vi "In Place_Unwired Terminals.vi"(8 "error in":errorcluster, 11 "In Place Node":refnum<vi>) -> (0 "error out":errorcluster, 1 "Unwired Indices For Removal":u32[](array[numeric]), 2 "Unwired Indices":u32[](array[numeric]), 3 "Output Terminals[]":refnum<vi>[](array[refnum]), 4 "Unwired?":bool[](array[boolean]))   [LabVIEW 2023]
doc: "Returns list of unwired terminals, and a separate list of those the can be removed. The latter will be different if all terminals are unwired, because you cannot remove *all* unwired terminals from the node.\n\nThe Unwired boolean array has one element per input/ouput terminal in inplace node."
panel:
  # "one element per terminal in node"
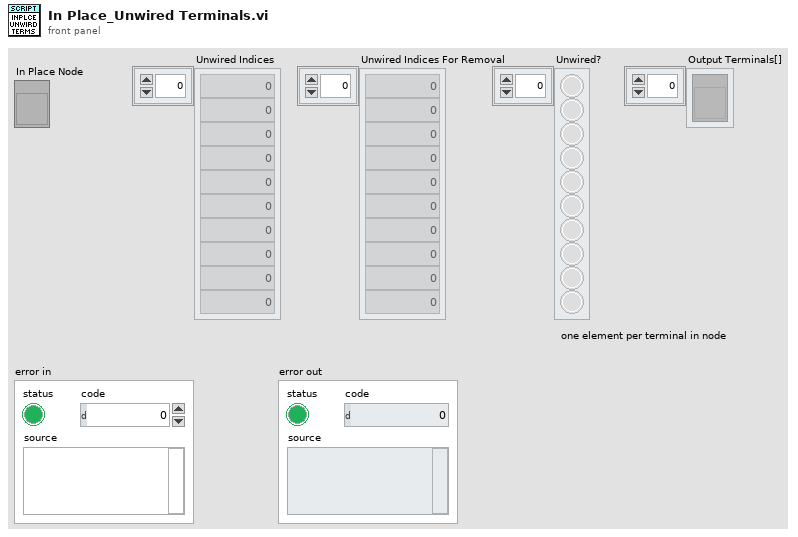
[diagram p1: front panel]
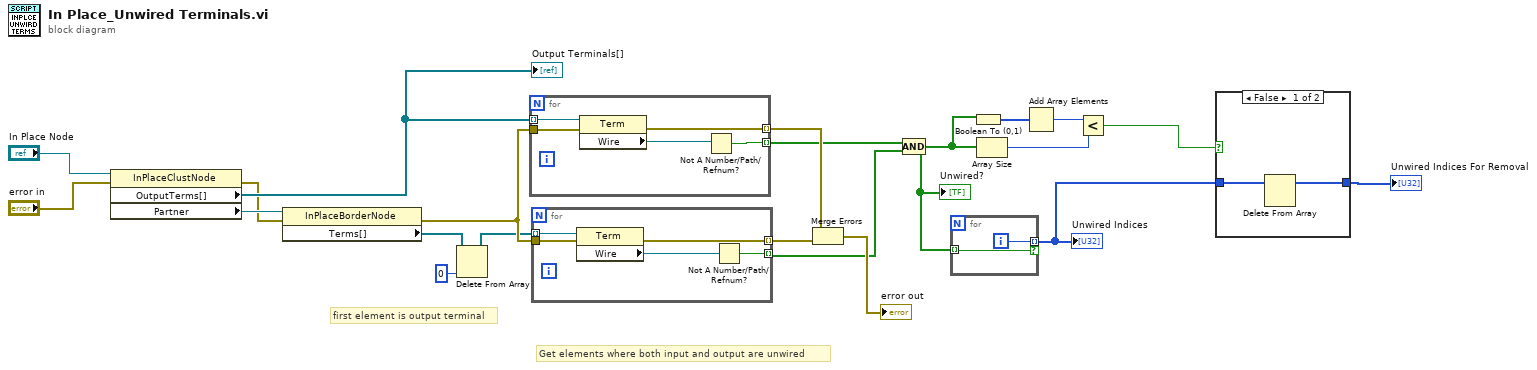
[diagram p0: block diagram]
diagram:
  # "first element is output terminal"
  # "Get elements where both input and output are unwired"
  n1 = property class="InPlaceClustNode"(reference="In Place Node", error in="error in") -> (error out=w15:errorcluster, "OutputTerms[]"=w19:refnum<vi>[], "Partner"=w21:refnum<vi>)  [unwired: 1 out]
  "Output Terminals[]" <- w19
  n2 = property class="InPlaceBorderNode"(reference=w21, error in=w15) -> (error out=w14:errorcluster, "Terms[]"=w5:refnum<vi>[])  [unwired: 1 out]
  n3 = Delete From Array(array=w5, index=0) -> (array with subset deleted=w4:refnum<vi>[])  [unwired: 1 in, 1 out]
  n4 = for {
    tunnel: [w22] -> w8 mode=indexing
    tunnel: w19 -> [w26] mode=indexing
    tunnel: w14 -> [w25]
    tunnel: [w24] -> w12 mode=indexing
    n5 = property class="Term"(reference=w26, error in=w25) -> (error out=w24:errorcluster, "Wire"=w23:refnum<vi>)  [unwired: 1 out]
    n6 = Not A Number/Path/Refnum?(number/path/refnum=w23) -> (NaN/Path/Refnum?=w22:bool)
  }
  n7 = for {
    tunnel: w4 -> [w31] mode=indexing
    tunnel: [w28] -> w7 mode=indexing
    tunnel: w14 -> [w30]
    tunnel: [w29] -> w13 mode=indexing
    n8 = property class="Term"(reference=w31, error in=w30) -> (error out=w29:errorcluster, "Wire"=w27:refnum<vi>)  [unwired: 1 out]
    n9 = Not A Number/Path/Refnum?(number/path/refnum=w27) -> (NaN/Path/Refnum?=w28:bool)
  }
  n10 = Merge Errors(w12, w13) -> (→"error out":errorcluster)
  n11 = Compound Arithmetic op=AND(w8, w7) -> (w17:bool[])
  "Unwired?" <- w17
  n12 = for {
    tunnel: w17 -> [w32] mode=indexing
    tunnel: [w33] -> w9 mode=indexing if=w32
    i -> [w33]
  }
  "Unwired Indices" <- w9
  n13 = Boolean To (0,1)(Boolean=w17) -> (0, 1=w18:i16[])
  n14 = Array Size(array=w17) -> (size(s)=w2:i32)
  n15 = Add Array Elements(numeric array=w18) -> (sum=w3:i16)
  n16 = Less?(x=w3, y=w2) -> (x < y?=w1:bool)
  n17 = case shown="False" w1 {
    tunnel: w9 -> [w35 w36]
    tunnel: [w34 w36] -> w10
    frame False {
      n18 = Delete From Array(array=w35) -> (array with subset deleted=w34:i32[])  [unwired: 2 in, 1 out]
    }
    frame True {
    }
  }
  "Unwired Indices For Removal" <- w10
